vi "OSC_xuanshaowen.vi"() -> ()   [LabVIEW 2012]
uses:
  <vilib>/Utility/miscctls.llb/LVTextColorsTypeDef.ctl
  <vilib>/Utility/miscctls.llb/LVForegroundBackgroundColorsTypeDef.ctl
  GlobalVariable.vi
panel:
  in  "选项卡控件":T1(tab)
  in  "开始":bool
  in  "停止":bool
  in  "AutoScale":bool
  in  "sample mode":u16(ring)=10178 caption="Acquisition Mode" items=["有限采样"=10178, "连续采样"=10123]
  in  "TriggleSetting":T2={"Type"=enum."Immediate", "Source"="", "Horizontal Position (%)"=0.5, "slope"=10280, "level"=0.0} {"level" step=0.01 format="%0.2f"; "slope" items=["上升"=10280, "下降"=10171]; "Horizontal Position (%)" scale=0.0..1.0}
  in  "TimeBase":cluster{"Time/Div":dbl}={"Time/Div"=0.001} {"Time/Div" scale=5e-06..0.2}
  in  "Channel Setting 0":T3={"physical channels"="", "Enable"=TRUE, "Coupling"=enum."DC", "    Scale\n  Volts/Div  "=0.5, "    Vertical\nPosition (Div)"=0.0, "Meas Range"=10.0} {"Meas Range" items=["-0.1 V~+0.1 V"=0.1, "-0.2 V~0.2 V"=0.2, "-0.5 V~+0.5 V"=0.5, "-1 V~+1 V"=1.0, "-2 V~+2 V"=2.0, "-5 V~+5 V"=5.0, "-10 V~+10 V"=10.0]; "Vertical\nPosition (Div)" min=-5.0 max=5.0 step=0.01 scale=-5.0..5.0 scale format="%.2f"; "Scale\n  Volts/Div" scale=0.01..20.0}
  in  "Channel Setting 1":T3={"physical channels"="", "Enable"=FALSE, "Coupling"=enum."DC", "    Scale\n  Volts/Div  "=0.5, "    Vertical\nPosition (Div)"=0.0, "Meas Range"=10.0} {"Meas Range" items=["-0.1 V~+0.1 V"=0.1, "-0.2 V~0.2 V"=0.2, "-0.5 V~+0.5 V"=0.5, "-1 V~+1 V"=1.0, "-2 V~+2 V"=2.0, "-5 V~+5 V"=5.0, "-10 V~+10 V"=10.0]; "Vertical\nPosition (Div)" min=-5.0 max=5.0 step=0.01 scale=-5.0..5.0 scale format="%.2f"; "Scale\n  Volts/Div" scale=0.01..20.0}
  out "Some Information":T4={"设计者："="宣劭文（文少轩）", "指导教师："="侯成刚", "单位："="西安交通大学", "设计说明："="      该示波器是设计者的一门实验课程的大作业，分享仅作学习交流用，请勿用于商业用途，转载请说明出处，请务必保留原作信息。\n\n      示波器的性能指标是基于NI的ELVISmx而确定的，具体见附件中的设计说明文档。\n\n      如有问题，欢迎来信交流。\n", "联系方式："="swxuan@live.com"}
  out "SampleRate:":string
  in  "Cursors":T5={"Cursors On"=FALSE, "Cursor 1"=FALSE, "CurChan1 1"=0, "Cursor 2"=FALSE, "CurChan1 2"=1} {"CurChan1 2" items=["CH1", "CH2"]; "CurChan1 1" items=["CH1", "CH2"]}
  in  "Meas On/Off":cluster{"CH0 Meas":bool, "CH1 Meas":bool}
  out "Cursor":string
  out "CH1 Meas":string
  out "CH0 Meas":string
  out "波形图":waveform(dbl)[](graph)
  # "Trigger"
  # "Timebase"
  # "Channel 0 Settings"
  # "Channel 1 Settings"
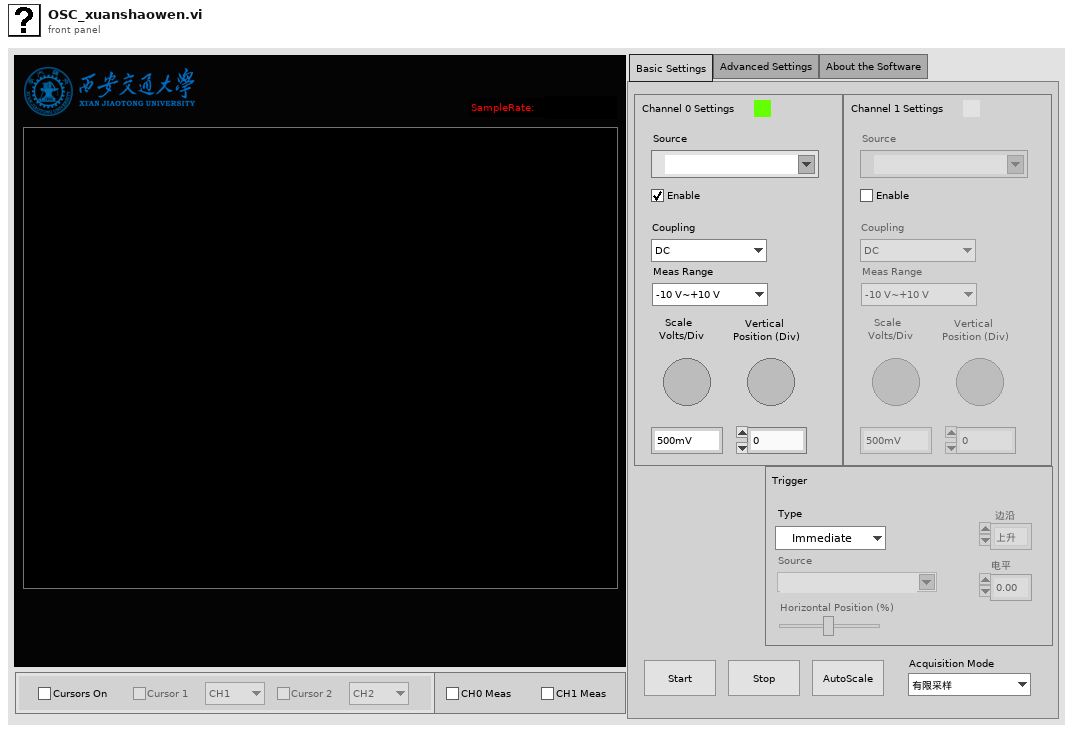
[diagram p1: front panel]
types:
  T1 = enum32{"Basic Settings", "Advanced Settings", "About the Software"}
  T2 = cluster{"Type":enum16{"Immediate", "Digital", "Edge"}, "Source":string, "Horizontal Position (%)":dbl, "slope":i32, "level":dbl}
  T3 = cluster{"physical channels":tag, "Enable":bool, "Coupling":enum16{"DC", "AC"}, "    Scale\n  Volts/Div  ":dbl, "    Vertical\nPosition (Div)":dbl, "Meas Range":dbl}
  T4 = cluster{"设计者：":string, "指导教师：":string, "单位：":string, "设计说明：":string, "联系方式：":string}
  T5 = cluster{"Cursors On":bool, "Cursor 1":bool, "CurChan1 1":u16, "Cursor 2":bool, "CurChan1 2":u16}
  T6 = typedef "LVForegroundBackgroundColorsTypeDef.ctl" = cluster{"Foreground Color":u32, "Background Color":u32}
  T7 = typedef "LVTextColorsTypeDef.ctl" = cluster{"Text Color":u32, "Background Color":u32}
  T8 = enum8{"Enabled", "Disabled", "Disabled and Grayed Out"}
  T9 = cluster{"数值输入控件":dbl, "最大值":dbl, "增量":dbl, "数值输入控件":dbl, "数值输入控件":dbl}
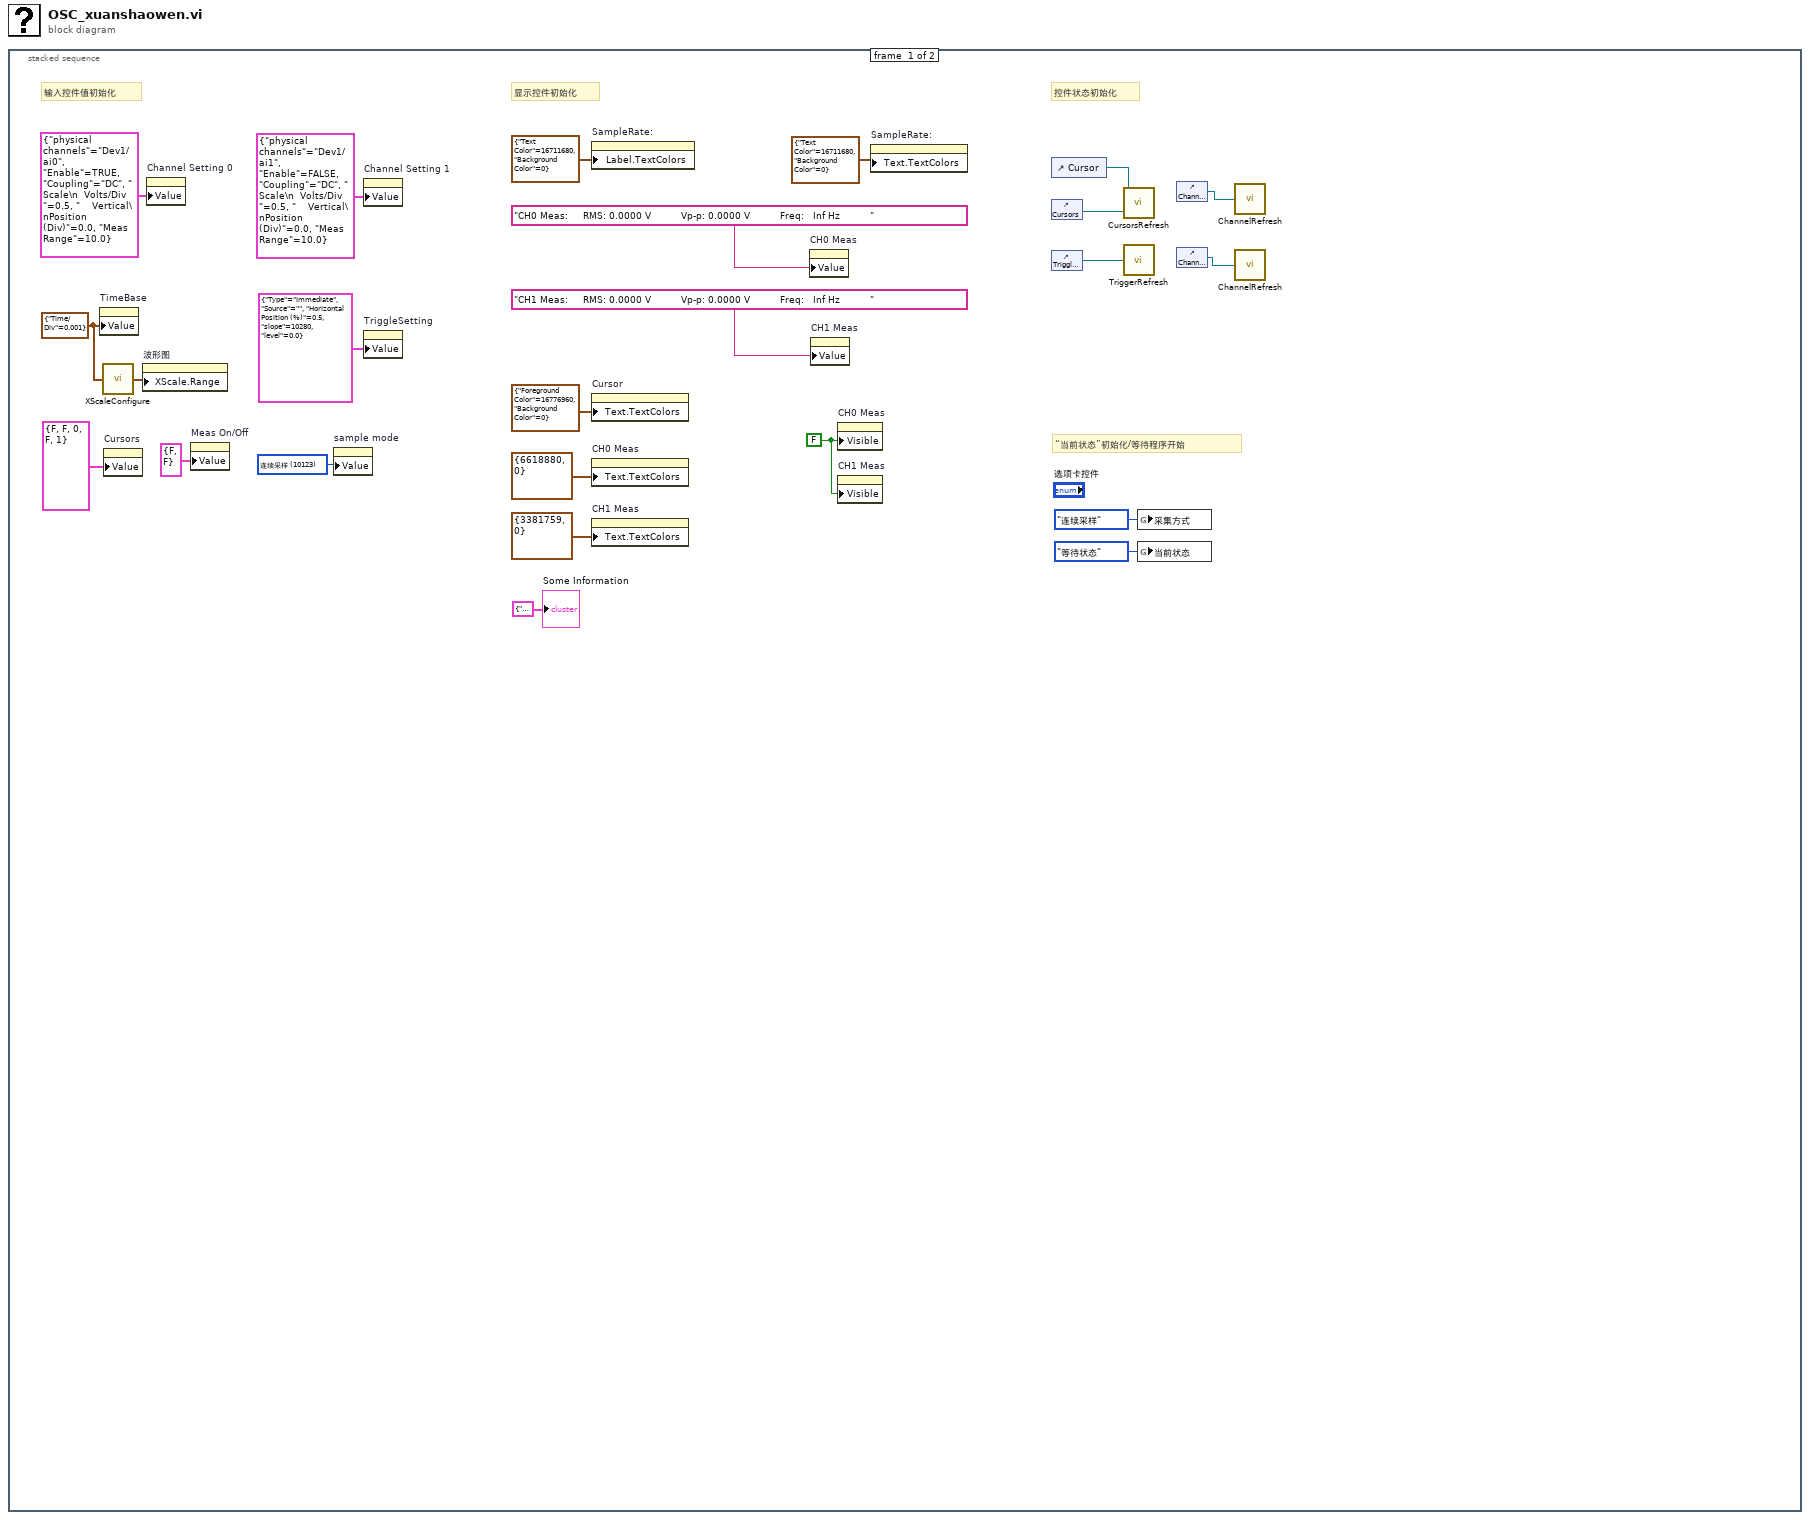
[diagram p0: block diagram]
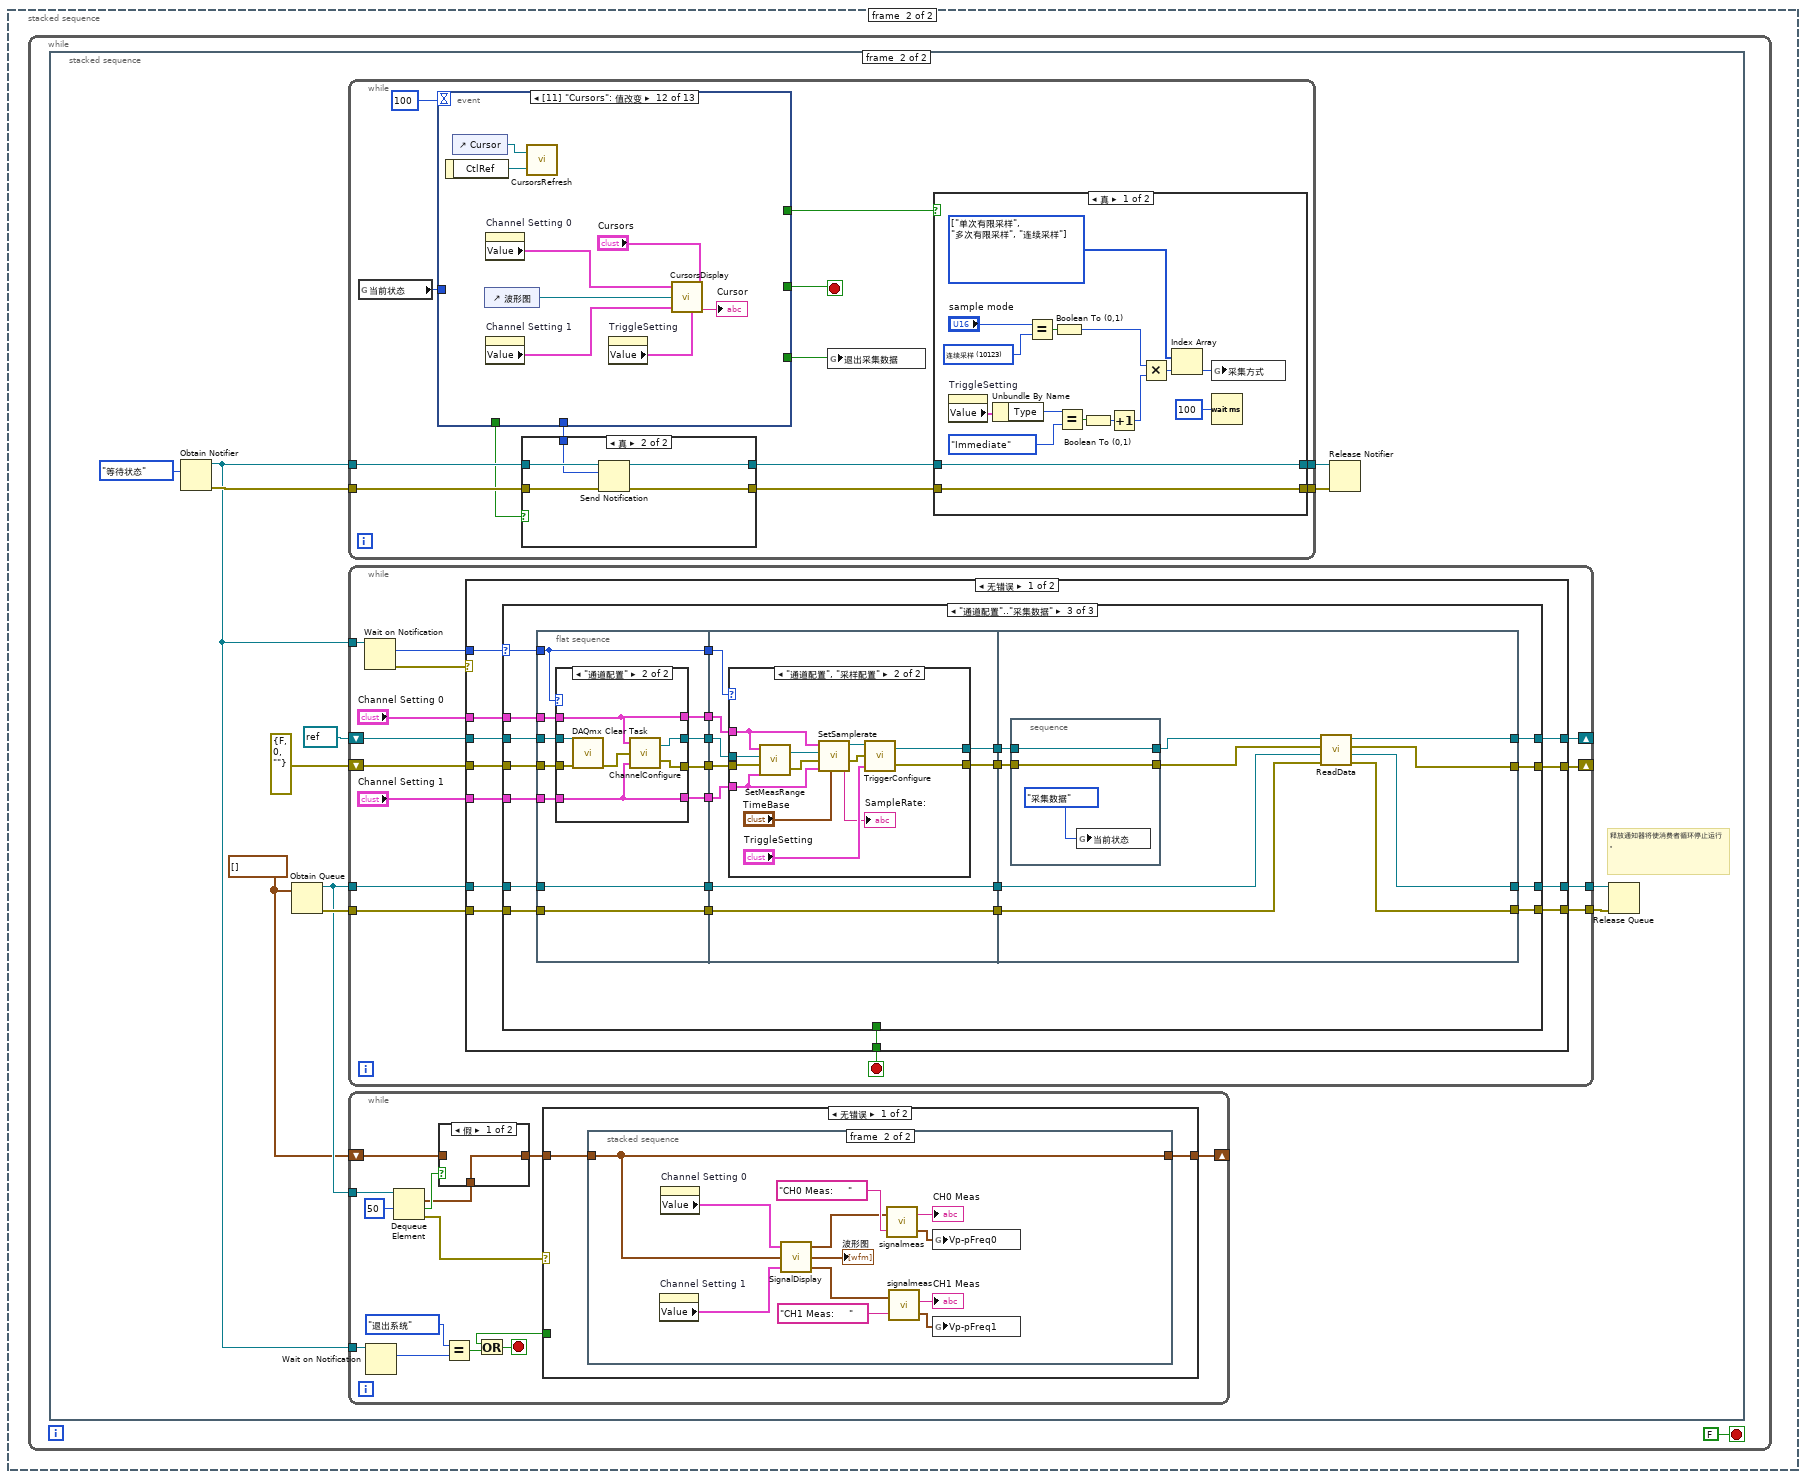
[diagram p2: hidden frame]
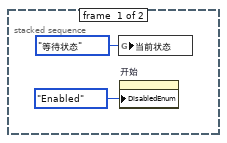
[diagram p3: hidden frame]
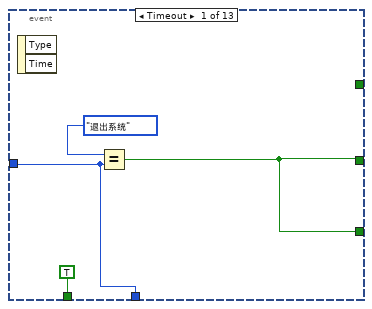
[diagram p5: hidden frame]
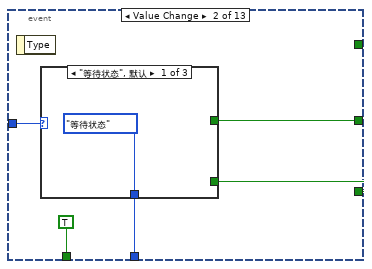
[diagram p6: hidden frame]
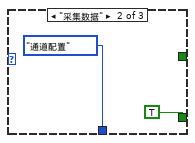
[diagram p7: hidden frame]
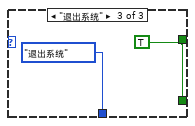
[diagram p8: hidden frame]
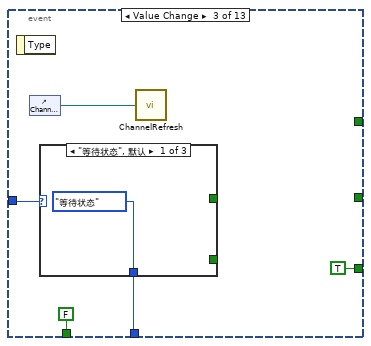
[diagram p9: hidden frame]
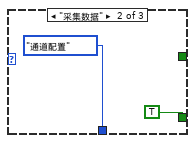
[diagram p10: hidden frame]
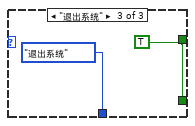
[diagram p11: hidden frame]
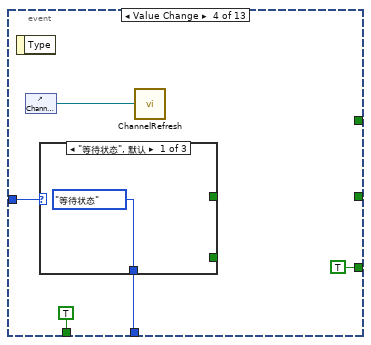
[diagram p12: hidden frame]
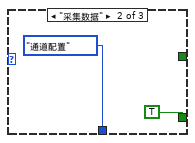
[diagram p13: hidden frame]
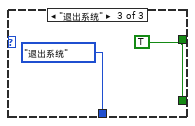
[diagram p14: hidden frame]
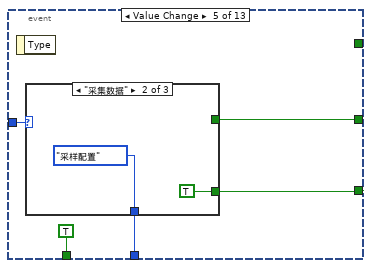
[diagram p15: hidden frame]
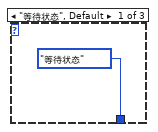
[diagram p16: hidden frame]
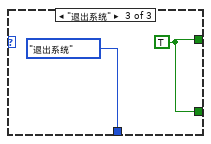
[diagram p17: hidden frame]
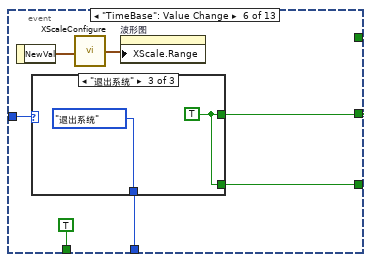
[diagram p18: hidden frame]
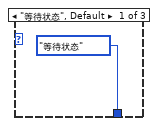
[diagram p19: hidden frame]
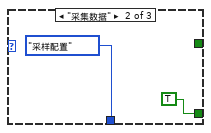
[diagram p20: hidden frame]
diagram:
  n1 = stacked-sequence {
    frame #0 {
      w2 = FALSE ("可见")
      w8 = u16 10123 items=["有限采样"=10178, "连续采样"=10123] ("sample mode")
      w22 = cluster{"Time/Div":dbl} {"Time/Div"=0.001} ("TimeBase")
      # "控件状态初始化"
      # "“当前状态”初始化/等待程序开始"
      # "显示控件初始化"
      # "输入控件值初始化"
      n2 = property on="TimeBase" class="Clust (严格)"("Value"=w22) -> ()  [unwired: 2 in, 2 out]
      n3 = call "XScaleConfigure.vi"("TimeBase"=w22) -> ("X坐标范围"=w21:T9)
      n4 = property on="Cursors" class="Clust (严格)"("Value"=T5 {"Cursors On"=FALSE, "Cursor 1"=FALSE, "CurChan1 1"=0, "Cursor 2"=FALSE, "CurChan1 2"=1} ("Cursors")) -> ()  [unwired: 2 in, 2 out]
      n5 = property on="波形图" class="WFGraph (严格)"("XScale.Range"=w21) -> ()  [unwired: 2 in, 2 out]
      n6 = property on="Channel Setting 0" class="Clust (严格)"("Value"=T3 {"physical channels"="Dev1/ai0", "Enable"=TRUE, "Coupling"=enum."DC", "    Scale\n  Volts/Div  "=0.5, "    Vertical\nPosition (Div)"=0.0, "Meas Range"=10.0} ("Channel Setting 0")) -> ()  [unwired: 2 in, 2 out]
      n7 = property on="Meas On/Off" class="Clust (严格)"("Value"=cluster{"CH0 Meas":bool, "CH1 Meas":bool} {"CH0 Meas"=FALSE, "CH1 Meas"=FALSE} ("Meas On/Off")) -> ()  [unwired: 2 in, 2 out]
      n8 = property on="sample mode" class="Ring (严格)"("Value"=w8) -> ()  [unwired: 2 in, 2 out]
      n9 = property on="Channel Setting 1" class="Clust (严格)"("Value"=T3 {"physical channels"="Dev1/ai1", "Enable"=FALSE, "Coupling"=enum."DC", "    Scale\n  Volts/Div  "=0.5, "    Vertical\nPosition (Div)"=0.0, "Meas Range"=10.0} ("Channel Setting 0")) -> ()  [unwired: 2 in, 2 out]
      n10 = property on="TriggleSetting" class="Clust (严格)"("Value"=T2 {"Type"=enum."Immediate", "Source"="", "Horizontal Position (%)"=0.5, "slope"=10280, "level"=0.0} ("TriggleSetting")) -> ()  [unwired: 2 in, 2 out]
      n11 = property on="SampleRate:" class="Str"("Label.TextColors"=T7 {"Text Color"=16711680, "Background Color"=0} ("标签.文本颜色")) -> ()  [unwired: 2 in, 2 out]
      n12 = property on="Cursor" class="Str"("Text.TextColors"=T6 {"Foreground Color"=16776960, "Background Color"=0} ("文本.颜色")) -> ()  [unwired: 2 in, 2 out]
      n13 = property on="CH0 Meas" class="Str"("Text.TextColors"=T7 {"Text Color"=6618880, "Background Color"=0} ("文本.文本颜色")) -> ()  [unwired: 2 in, 2 out]
      n14 = property on="CH1 Meas" class="Str"("Text.TextColors"=T7 {"Text Color"=3381759, "Background Color"=0} ("文本.文本颜色")) -> ()  [unwired: 2 in, 2 out]
      n15 = property on="CH0 Meas" class="Str"("Value"="CH0 Meas:     RMS: 0.0000 V          Vp-p: 0.0000 V          Freq:   Inf Hz          " ("CH0 Meas")) -> ()  [unwired: 2 in, 2 out]
      n16 = property on="CH1 Meas" class="Str"("Value"="CH1 Meas:     RMS: 0.0000 V          Vp-p: 0.0000 V          Freq:   Inf Hz          " ("CH1 Meas")) -> ()  [unwired: 2 in, 2 out]
      n17 = property on="CH0 Meas" class="Str"("Visible"=w2) -> ()  [unwired: 2 in, 2 out]
      n18 = property on="CH1 Meas" class="Str"("Visible"=w2) -> ()  [unwired: 2 in, 2 out]
      n19 = property on="SampleRate:" class="Str"("Text.TextColors"=T7 {"Text Color"=16711680, "Background Color"=0} ("数值文本.文本颜色")) -> ()  [unwired: 2 in, 2 out]
      n20 = control-ref of="Cursor"() -> (w9:refnum<vi>)
      n21 = control-ref of="Cursors"() -> (w10:refnum<vi>)
      n22 = control-ref of="TriggleSetting"() -> (w7:refnum<vi>)
      n23 = call "CursorsRefresh.vi"("Cursors簇句柄引用"=w10, "Cursor字符串句柄引用"=w9) -> ()  [unwired: 2 in]
      n24 = call "TriggerRefresh.vi"("TriggerSetting引用句柄"=w7) -> ()
      n25 = global write "GlobalVariable.vi" "采集方式"(enum16{"单次有限采样", "多次有限采样", "连续采样"}."连续采样" ("采集方式")) -> ()
      n26 = global write "GlobalVariable.vi" "当前状态"(enum16{"等待状态", "采集数据", "退出系统"}."等待状态" ("当前状态")) -> ()
      n27 = control-ref of="Channel Setting 0"() -> (w6:refnum<vi>)
      n28 = control-ref of="Channel Setting 1"() -> (w5:refnum<vi>)
      n29 = call "ChannelRefresh.vi"("Channel Setting 引用句柄"=w6) -> ()
      n30 = call "ChannelRefresh.vi"("Channel Setting 引用句柄"=w5) -> ()
      "Some Information" <- T4 {"设计者："="宣劭文（文少轩）", "指导教师："="侯成刚", "单位："="西安交通大学", "设计说明："="      该示波器是设计者的一门实验课程的大作业，分享仅作学习交流用，请勿用于商业用途，转载请说明出处，请务必保留原作信息。\n\n      示波器的性能指标是基于NI的ELVISmx而确定的，具体见附件中的设计说明文档。\n\n      如有问题，欢迎来信交流。\n", "联系方式："="swxuan@live.com"} ("Some Information")
    }
    frame #1 {
      n31 = while {
        stop <- FALSE stop-if-true
        n32 = stacked-sequence {
          frame #0 {
            n33 = global write "GlobalVariable.vi" "当前状态"(enum16{"等待状态", "采集数据", "退出系统"}."等待状态" ("当前状态")) -> ()
            n34 = property on="开始" class="Bool"("DisabledEnum"=T8."Enabled" ("禁用")) -> ()  [unwired: 2 in, 2 out]
          }
          frame #1 {
            w28 = waveform(dbl)[] [] ("data")
            # "释放通知器将使消费者循环停止运行。"
            n35 = Obtain Notifier(notification data type=enum16{"等待状态", "通道配置", "采样配置", "采集数据", "退出系统"}."等待状态" ("当前状态")) -> (notifier out=w31:refnum<notifier>, error out=w35:errorcluster)  [unwired: 2 in, 2 out]
            n36 = Obtain Queue(element data type=w28) -> (queue out=w36:refnum<queue>, error out=w39:errorcluster)  [unwired: 4 in, 1 out]
            n37 = while {
              tunnel: w31 -> [w52]
              tunnel: w35 -> [w51]
              tunnel: [w48] -> w34
              tunnel: [w47] -> w33
              stop <- w42 stop-if-true
              n38 = global read "GlobalVariable.vi" "当前状态"() -> (w46:enum16{"等待状态", "采集数据", "退出系统"})
              n39 = event shown="[11] \"Cursors\": 值改变" {
                selector: _ -> [_ _ _ _ _ _ _ _ _ _ _ _ _]
                dyn-events: _ -> [_ _ _ _ _ _ _ _ _ _ _ _ _]
                timeout: 100 -> [_ _ _ _ _ _ _ _ _ _ _ _ _]
                tunnel: w46 -> [w72 w79 w86 w96 w109 w120 w132 _ _ w149 w166 _ _]
                tunnel: [w72 w78 w85 w95 w108 w119 w131 enum16{"等待状态", "通道配置", "采样配置", "采集数据", "退出系统"}."通道配置" ("当前状态") enum16{"等待状态", "通道配置", "采样配置", "采集数据", "退出系统"}."退出系统" ("当前状态") w147 w165 _ _] -> w44
                tunnel: [TRUE TRUE FALSE TRUE TRUE TRUE TRUE TRUE TRUE w148 TRUE _ _] -> w43
                tunnel: [w71 w76 _ _ w106 w117 w129 _ w142 w145 w163 _ _] -> w42
                tunnel: [w71 w75 TRUE TRUE w105 w115 w128 _ w142 w146 w162 _ _] -> w41
                tunnel: [_ _ _ _ _ _ TRUE _ _ _ TRUE _ _] -> w40
                event Timeout {
                  n40 = event-data() -> ()  [unwired: 1 in, 2 out]
                  n41 = Equal?(x=enum16{"等待状态", "采集数据", "退出系统"}."退出系统", y=w72) -> (x = y?=w71:bool)
                }
                event "Channel Setting 0.physical channels", "Channel Setting 1.physical channels": Value Change {
                  n42 = event-data() -> ()  [unwired: 1 in, 1 out]
                  n43 = case shown="\"等待状态\", 默认" w79 {
                    tunnel: [enum16{"等待状态", "通道配置", "采样配置", "采集数据", "退出系统"}."等待状态" ("当前状态") enum16{"等待状态", "通道配置", "采样配置", "采集数据", "退出系统"}."通道配置" ("当前状态") enum16{"等待状态", "通道配置", "采样配置", "采集数据", "退出系统"}."退出系统" ("当前状态")] -> w78
                    tunnel: [_ TRUE w83] -> w75
                    tunnel: [_ _ w83] -> w76
                    frame "等待状态", Default {
                    }
                    frame "采集数据" {
                    }
                    frame "退出系统" {
                      w83 = TRUE
                    }
                  }
                }
                event "Channel Setting 0.Enable": Value Change {
                  n44 = event-data() -> ()  [unwired: 1 in, 1 out]
                  n45 = control-ref of="Channel Setting 0"() -> (w89:refnum<vi>)
                  n46 = case shown="\"等待状态\", 默认" w86 {
                    tunnel: [enum16{"等待状态", "通道配置", "采样配置", "采集数据", "退出系统"}."等待状态" ("当前状态") enum16{"等待状态", "通道配置", "采样配置", "采集数据", "退出系统"}."通道配置" ("当前状态") enum16{"等待状态", "通道配置", "采样配置", "采集数据", "退出系统"}."退出系统" ("当前状态")] -> w85
                    tunnel: [_ TRUE w93] -> _
                    tunnel: [_ _ w93] -> _
                    frame "等待状态", Default {
                    }
                    frame "采集数据" {
                    }
                    frame "退出系统" {
                      w93 = TRUE
                    }
                  }
                  n47 = call "ChannelRefresh.vi"("Channel Setting 引用句柄"=w89) -> ()
                }
                event "Channel Setting 1.Enable": Value Change {
                  n48 = event-data() -> ()  [unwired: 1 in, 1 out]
                  n49 = control-ref of="Channel Setting 1"() -> (w99:refnum<vi>)
                  n50 = case shown="\"等待状态\", 默认" w96 {
                    tunnel: [enum16{"等待状态", "通道配置", "采样配置", "采集数据", "退出系统"}."等待状态" ("当前状态") enum16{"等待状态", "通道配置", "采样配置", "采集数据", "退出系统"}."通道配置" ("当前状态") enum16{"等待状态", "通道配置", "采样配置", "采集数据", "退出系统"}."退出系统" ("当前状态")] -> w95
                    tunnel: [_ TRUE w103] -> _
                    tunnel: [_ _ w103] -> _
                    frame "等待状态", Default {
                    }
                    frame "采集数据" {
                    }
                    frame "退出系统" {
                      w103 = TRUE
                    }
                  }
                  n51 = call "ChannelRefresh.vi"("Channel Setting 引用句柄"=w99) -> ()
                }
                event "Channel Setting 0.Meas Range", "Channel Setting 1.Meas Range": Value Change {
                  n52 = event-data() -> ()  [unwired: 1 in, 1 out]
                  n53 = case shown="\"采集数据\"" w109 {
                    tunnel: [enum16{"等待状态", "通道配置", "采样配置", "采集数据", "退出系统"}."等待状态" ("当前状态") enum16{"等待状态", "通道配置", "采样配置", "采集数据", "退出系统"}."采样配置" ("当前状态") enum16{"等待状态", "通道配置", "采样配置", "采集数据", "退出系统"}."退出系统" ("当前状态")] -> w108
                    tunnel: [_ TRUE w114] -> w105
                    tunnel: [_ _ w114] -> w106
                    frame "等待状态", Default {
                    }
                    frame "采集数据" {
                    }
                    frame "退出系统" {
                      w114 = TRUE
                    }
                  }
                }
                event "TimeBase": Value Change {
                  n54 = event-data() -> ("NewVal"=w121:cluster{"Time/Div":dbl})  [unwired: 1 in]
                  n55 = case shown="\"退出系统\"" w120 {
                    tunnel: [enum16{"等待状态", "通道配置", "采样配置", "采集数据", "退出系统"}."等待状态" ("当前状态") enum16{"等待状态", "通道配置", "采样配置", "采集数据", "退出系统"}."采样配置" ("当前状态") enum16{"等待状态", "通道配置", "采样配置", "采集数据", "退出系统"}."退出系统" ("当前状态")] -> w119
                    tunnel: [_ _ w125] -> w117
                    tunnel: [_ TRUE w125] -> w115
                    frame "等待状态", Default {
                    }
                    frame "采集数据" {
                    }
                    frame "退出系统" {
                      w125 = TRUE
                    }
                  }
                  n56 = call "XScaleConfigure.vi"("TimeBase"=w121) -> ("X坐标范围"=w116:T9)
                  n57 = property on="波形图" class="WFGraph (严格)"("XScale.Range"=w116) -> ()  [unwired: 2 in, 2 out]
                }
                event "TriggleSetting": Value Change {
                  n58 = event-data() -> ("CtlRef"=w133:refnum<vi>)  [unwired: 1 in]
                  n59 = case shown="\"退出系统\"" w132 {
                    tunnel: [enum16{"等待状态", "通道配置", "采样配置", "采集数据", "退出系统"}."等待状态" ("当前状态") enum16{"等待状态", "通道配置", "采样配置", "采集数据", "退出系统"}."采样配置" ("当前状态") enum16{"等待状态", "通道配置", "采样配置", "采集数据", "退出系统"}."退出系统" ("当前状态")] -> w131
                    tunnel: [_ TRUE w137] -> w128
                    tunnel: [_ _ w137] -> w129
                    frame "等待状态", Default {
                    }
                    frame "采集数据" {
                    }
                    frame "退出系统" {
                      w137 = TRUE
                    }
                  }
                  n60 = call "TriggerRefresh.vi"("TriggerSetting引用句柄"=w133) -> ()
                }
                event "开始": Value Change {
                  n61 = event-data() -> ()  [unwired: 1 in, 1 out]
                  n62 = property on="开始" class="Bool"("DisabledEnum"=T8."Disabled and Grayed Out" ("禁用")) -> ()  [unwired: 2 in, 2 out]
                }
                event "停止": Value Change {
                  w142 = TRUE
                  n63 = event-data() -> ()  [unwired: 1 in, 1 out]
                }
                event "AutoScale": Value Change {
                  n64 = event-data() -> ()  [unwired: 1 in, 1 out]
                  n65 = case shown="\"采集数据\"" w149 {
                    tunnel: [_ _ w158] -> w145
                    tunnel: [_ enum16{"等待状态", "通道配置", "采样配置", "采集数据", "退出系统"}."采样配置" ("当前状态") enum16{"等待状态", "通道配置", "采样配置", "采集数据", "退出系统"}."退出系统" ("当前状态")] -> w147
                    tunnel: [_ TRUE TRUE] -> w148
                    tunnel: [_ TRUE w158] -> w146
                    frame "等待状态", Default {
                    }
                    frame "采集数据" {
                      n66 = property on="Enable" class="Bool (严格)"() -> ("Value"=w157:bool)  [unwired: 2 in, 2 out]
                      n67 = property on="Enable" class="Bool (严格)"() -> ("Value"=w156:bool)  [unwired: 2 in, 2 out]
                      n68 = call "AutoScale.vi"("Channel 1 Enable"=w156, "Channel 0 Enable"=w157) -> ("Scale\n  Volts/Div 1"=w153:dbl, "Time/Div"=w154:dbl, "Scale\n  Volts/Div 0"=w155:dbl)  [unwired: 2 in]
                      n69 = property on="Time/Div" class="Knob (严格)"("Value"=w154) -> ()  [unwired: 2 in, 2 out]
                      n70 = property on="Scale\n  Volts/Div" class="Knob (严格)"("Value"=w155) -> ()  [unwired: 2 in, 2 out]
                      n71 = property on="Scale\n  Volts/Div" class="Knob (严格)"("Value"=w153) -> ()  [unwired: 2 in, 2 out]
                    }
                    frame "退出系统" {
                      w158 = TRUE
                    }
                  }
                }
                event "sample mode": Value Change {
                  n72 = event-data() -> ()  [unwired: 1 in, 1 out]
                  n73 = case shown="\"等待状态\", 默认" w166 {
                    tunnel: [enum16{"等待状态", "通道配置", "采样配置", "采集数据", "退出系统"}."等待状态" ("当前状态") enum16{"等待状态", "通道配置", "采样配置", "采集数据", "退出系统"}."采样配置" ("当前状态") enum16{"等待状态", "通道配置", "采样配置", "采集数据", "退出系统"}."退出系统" ("当前状态")] -> w165
                    tunnel: [_ TRUE w170] -> w162
                    tunnel: [_ _ w170] -> w163
                    frame "等待状态", Default {
                    }
                    frame "采集数据" {
                    }
                    frame "退出系统" {
                      w170 = TRUE
                    }
                  }
                }
                event "Cursors": Value Change {
                  n74 = event-data() -> ("CtlRef"=w179:refnum<vi>)  [unwired: 1 in]
                  n75 = control-ref of="Cursor"() -> (w178:refnum<vi>)
                  n76 = control-ref of="波形图"() -> (w176:refnum<vi>)
                  n77 = property on="Channel Setting 0" class="Clust (严格)"() -> ("Value"=w177:T3)  [unwired: 2 in, 2 out]
                  n78 = property on="Channel Setting 1" class="Clust (严格)"() -> ("Value"=w175:T3)  [unwired: 2 in, 2 out]
                  n79 = call "CursorsRefresh.vi"("Cursors簇句柄引用"=w179, "Cursor字符串句柄引用"=w178) -> ()  [unwired: 2 in]
                  n80 = property on="TriggleSetting" class="Clust (严格)"() -> ("Value"=w174:T2)  [unwired: 2 in, 2 out]
                  n81 = call "CursorsDisplay.vi"("Channel Setting 0"=w177, "波形图引用句柄"=w176, "Channel Setting 1"=w175, "Cursors"="Cursors", "TriggleSetting"=w174) -> ("Cursor"=→"Cursor":string)  [unwired: 5 in]
                }
                event "Meas On/Off": Value Change {
                  n82 = event-data() -> ("NewVal"=w180:cluster{"CH0 Meas":bool, "CH1 Meas":bool})  [unwired: 1 in]
                  n83 = Unbundle By Name(w180) -> ("CH0 Meas"=w181:bool, "CH1 Meas"=w182:bool)
                  n84 = property on="CH1 Meas" class="Str"("Visible"=w182) -> ()  [unwired: 2 in, 2 out]
                  n85 = property on="CH0 Meas" class="Str"("Visible"=w181) -> ()  [unwired: 2 in, 2 out]
                }
              }
              n86 = case shown="真" w43 {
                tunnel: w52 -> [w183 w189]
                tunnel: [w184 w188] -> w49
                tunnel: w51 -> [w184 w187]
                tunnel: [w183 w186] -> w50
                tunnel: w44 -> [_ w185]
                frame False {
                }
                frame True {
                  n87 = Send Notification(notification=w185, notifier=w189, error in (no error)=w187) -> (notifier out=w186:refnum<notifier>, error out=w188:errorcluster)
                }
              }
              n88 = global write "GlobalVariable.vi" "退出采集数据"(w41) -> ()
              n89 = case shown="真" w40 {
                tunnel: w50 -> [w57 w70]
                tunnel: w49 -> [w56 w69]
                tunnel: [w57 w70] -> w48
                tunnel: [w56 w69] -> w47
                frame True {
                  w59 = u16 10123 items=["有限采样"=10178, "连续采样"=10123] ("sample mode")
                  w68 = enum16{"单次有限采样", "多次有限采样", "连续采样"}[] [enum."单次有限采样", enum."多次有限采样", enum."连续采样"] items=["单次有限采样", "多次有限采样", "连续采样"]
                  n90 = property on="TriggleSetting" class="Clust (严格)"() -> ("Value"=w63:T2)  [unwired: 2 in, 2 out]
                  n91 = Unbundle By Name(w63) -> ("Type"=w62:enum16{"Immediate", "Digital", "Edge"})
                  n92 = Equal?(x="sample mode", y=w59) -> (x = y?=w60:bool)
                  n93 = Boolean To (0,1)(Boolean=w60) -> (0, 1=w67:i16)
                  n94 = Equal?(x=w62, y=enum16{"Immediate", "Digital", "Edge"}."Immediate") -> (x = y?=w64:bool)
                  n95 = Boolean To (0,1)(Boolean=w64) -> (0, 1=w65:i16)
                  n96 = Increment(x=w65) -> (x+1=w66:i16)
                  n97 = Multiply(x=w67, y=w66) -> (x*y=w54:i16)
                  n98 = Index Array(array=w68, index=w54) -> (element=w55:enum16{"单次有限采样", "多次有限采样", "连续采样"})
                  n99 = global write "GlobalVariable.vi" "采集方式"(w55) -> ()
                  n100 = Wait (ms)(milliseconds to wait=u32 100 ("等待时间（毫秒）")) -> ()  [unwired: 1 out]
                }
                frame False {
                }
              }
            }
            n101 = while {
              tunnel: w36 -> [w241]
              tunnel: w39 -> [w240]
              tunnel: [w239] -> w38
              tunnel: [w238] -> w37
              tunnel: w31 -> [w237]
              shift-right: [w233] -> _
              shift-left: refnum<k21> refnum ("task out") -> [w234]
              shift-right: [w235] -> _
              shift-left: errorcluster {"status"=FALSE, "code"=0, "source"=""} ("error out") -> [w236]
              stop <- w230 stop-if-true
              n102 = Wait on Notification(notifier=w237) -> (notification=w232:enum16{"等待状态", "通道配置", "采样配置", "采集数据", "退出系统"}, error out=w231:errorcluster)  [unwired: 1 in, 4 out]
              n103 = case shown="无错误" w231 {
                tunnel: w241 -> [w253 w350]
                tunnel: w240 -> [w252 w349]
                tunnel: [w251 w350] -> w239
                tunnel: [w250 w349] -> w238
                tunnel: w236 -> [w249 w347]
                tunnel: [w248 w347] -> w235
                tunnel: w234 -> [w247 w348]
                tunnel: [w246 w348] -> w233
                tunnel: w232 -> [w244 _]
                tunnel: [w245 TRUE] -> w230
                tunnel: "Channel Setting 0" -> [w243 _]
                tunnel: "Channel Setting 1" -> [w242 _]
                frame No Error {
                  n104 = case shown="\"通道配置\"..\"采集数据\"" w244 {
                    selector: w244 -> [_ _ w286]
                    tunnel: w253 -> [w256 w261 w283]
                    tunnel: w252 -> [w255 w260 w282]
                    tunnel: [w256 w261 w281] -> w251
                    tunnel: [w255 w260 w280] -> w250
                    tunnel: w249 -> [w257 w262 w284]
                    tunnel: [w257 w262 w278] -> w248
                    tunnel: w247 -> [w258 w263 w285]
                    tunnel: [w258 w263 w279] -> w246
                    tunnel: [_ TRUE _] -> w245
                    tunnel: w243 -> [_ _ w271]
                    tunnel: w242 -> [_ _ w270]
                    frame "等待状态", Default {
                      n105 = Wait (ms)(milliseconds to wait=u32 50 ("等待时间（毫秒）")) -> ()  [unwired: 1 out]
                    }
                    frame "退出系统" {
                      n106 = global write "GlobalVariable.vi" "当前状态"(enum16{"等待状态", "采集数据", "退出系统"}."退出系统" ("当前状态")) -> ()
                    }
                    frame "通道配置".."采集数据" {
                      n107 = flat-sequence {
                        tunnel: w286 -> [w287]
                        tunnel: w285 -> [w297]
                        tunnel: [w293] -> w277
                        tunnel: w284 -> [w296]
                        tunnel: [w292] -> w276
                        tunnel: w283 -> [w295]
                        tunnel: [w295] -> w275
                        tunnel: w282 -> [w294]
                        tunnel: [w294] -> w274
                        tunnel: w271 -> [w291]
                        tunnel: w270 -> [w290]
                        tunnel: [w289] -> w269
                        tunnel: [w288] -> w268
                        tunnel: [w287] -> w267
                        tunnel: w277 -> [w317]
                        tunnel: w276 -> [w316]
                        tunnel: w275 -> [w315]
                        tunnel: [w315] -> w273
                        tunnel: w274 -> [w314]
                        tunnel: [w314] -> w272
                        tunnel: w269 -> [w313]
                        tunnel: w268 -> [w312]
                        tunnel: w267 -> [w311]
                        tunnel: [w310] -> w266
                        tunnel: [w309] -> w265
                        tunnel: w273 -> [w336]
                        tunnel: w272 -> [w335]
                        tunnel: [w334] -> w281
                        tunnel: [w333] -> w280
                        tunnel: [w340] -> w279
                        tunnel: [w339] -> w278
                        tunnel: w266 -> [w338]
                        tunnel: w265 -> [w337]
                        frame #0 {
                          n108 = case shown="\"通道配置\"" w287 {
                            tunnel: w297 -> [w301 w307]
                            tunnel: w296 -> [w300 w306]
                            tunnel: [w301 w305] -> w293
                            tunnel: [w300 w304] -> w292
                            tunnel: w291 -> [w299 w303]
                            tunnel: w290 -> [w298 w302]
                            tunnel: [w299 w303] -> w289
                            tunnel: [w298 w302] -> w288
                            frame "采样配置", "采集数据", Default {
                            }
                            frame "通道配置" {
                              n109 = call <vilib>:"DAQmx Clear Task.vi"("task in"=w307, "error in"=w306) -> ("error out"=w308:errorcluster)  [unwired: 13 in]
                              n110 = call "ChannelConfigure.vi"("Channel Setting 1"=w302, "Error In"=w308, "Channel Setting 0"=w303) -> ("Error Out"=w304:errorcluster, "Task Out"=w305:refnum<k21>)
                            }
                          }
                        }
                        frame #1 {
                          n111 = case shown="\"通道配置\", \"采样配置\"" w311 {
                            tunnel: w317 -> [w319 w328]
                            tunnel: w316 -> [w318 w327]
                            tunnel: w313 -> [_ w326]
                            tunnel: w312 -> [_ w325]
                            tunnel: [w319 w321] -> w310
                            tunnel: [w318 w320] -> w309
                            frame "采集数据", Default {
                            }
                            frame "通道配置", "采样配置" {
                              n112 = call "SetMeasRange.vi"("Channel Setting 1"=w325, "Error In"=w327, "Task In"=w328, "Channel Setting 0"=w326) -> ("Error Out"=w330:errorcluster, "Task Out"=w331:refnum<k21>)
                              n113 = call "SetSamplerate.vi"("TimeBase"="TimeBase", "Channel Setting 1"=w325, "Error In"=w330, "Task In"=w331, "Channel Setting 0"=w326) -> ("采样率"=→"SampleRate:":string, "Error Out"=w322:errorcluster, "Task Out"=w323:refnum<k21>)  [unwired: 2 in]
                              n114 = call "TriggerConfigure.vi"("TriggleSetting"="TriggleSetting", "Error In"=w322, "Task In"=w323) -> ("Error Out"=w320:errorcluster, "Task Out"=w321:refnum<k21>)
                            }
                          }
                        }
                        frame #2 {
                          n115 = stacked-sequence {
                            tunnel: [w345] -> w341
                            tunnel: w338 -> [w345]
                            tunnel: [w344] -> w342
                            tunnel: w337 -> [w344]
                            frame #0 {
                              n116 = global write "GlobalVariable.vi" "当前状态"(enum16{"等待状态", "采集数据", "退出系统"}."采集数据" ("当前状态")) -> ()
                            }
                          }
                          n117 = call "ReadData.vi"("错误输入（队列）"=w335, "队列输入"=w336, "错误输入（采集）"=w342, "Task In"=w341) -> ("错误输出（队列）"=w333:errorcluster, "队列输出"=w334:refnum<queue>, "错误输出（采集）"=w339:errorcluster, "Task Out"=w340:refnum<k21>)
                        }
                      }
                    }
                  }
                }
                frame Error {
                  n118 = global write "GlobalVariable.vi" "当前状态"(enum16{"等待状态", "采集数据", "退出系统"}."退出系统" ("当前状态")) -> ()
                }
              }
            }
            n119 = while {
              tunnel: w36 -> [w203]
              tunnel: w31 -> [w200]
              shift-right: [w190] -> _
              shift-left: w28 -> [w193]
              stop <- w202 stop-if-true
              n120 = Wait on Notification(notifier=w200) -> (notification=w198:enum16{"等待状态", "通道配置", "采样配置", "采集数据", "退出系统"})  [unwired: 1 in, 5 out]
              n121 = Dequeue Element(queue=w203, timeout in ms (-1)=50 ("超时毫秒(-1)")) -> (element=w192:waveform(dbl)[], timed out?=w194:bool, error out=w197:errorcluster)  [unwired: 1 in, 1 out]
              n122 = case shown="假" w194 {
                tunnel: w193 -> [_ w205]
                tunnel: w192 -> [w204 _]
                tunnel: [w204 w205] -> w191
                frame False {
                }
                frame True {
                }
              }
              n123 = Equal?(x=enum16{"等待状态", "通道配置", "采样配置", "采集数据", "退出系统"}."退出系统" ("当前状态"), y=w198) -> (x = y?=w201:bool)
              n124 = case shown="无错误" w197 {
                tunnel: [_ TRUE] -> w196
                tunnel: w191 -> [w207 _]
                tunnel: [w206 _] -> w190
                frame No Error {
                  n125 = stacked-sequence {
                    tunnel: w207 -> [_ w214]
                    tunnel: [_ w214] -> w206
                    frame #0 {
                      n126 = property on="Channel Setting 0" class="Clust (严格)"() -> ("Value"=w213:T3)  [unwired: 2 in, 2 out]
                      n127 = control-ref of="波形图"() -> (w211:refnum<vi>)
                      n128 = property on="Channel Setting 1" class="Clust (严格)"() -> ("Value"=w212:T3)  [unwired: 2 in, 2 out]
                      n129 = property on="TriggleSetting" class="Clust (严格)"() -> ("Value"=w208:T2)  [unwired: 2 in, 2 out]
                      n130 = property on="Cursors" class="Clust (严格)"() -> ("Value"=w209:T5)  [unwired: 2 in, 2 out]
                      n131 = call "CursorsDisplay.vi"("Channel Setting 0"=w213, "波形图引用句柄"=w211, "Channel Setting 1"=w212, "Cursors"=w209, "TriggleSetting"=w208) -> ("Cursor"=w210:string)  [unwired: 5 in]
                      n132 = property on="Cursor" class="Str"("Value"=w210) -> ()  [unwired: 2 in, 2 out]
                    }
                    frame #1 {
                      n133 = property on="Channel Setting 1" class="Clust (严格)"() -> ("Value"=w220:T3)  [unwired: 2 in, 2 out]
                      n134 = property on="Channel Setting 0" class="Clust (严格)"() -> ("Value"=w221:T3)  [unwired: 2 in, 2 out]
                      n135 = call "SignalDisplay.vi"("Channel Setting 1"=w220, "Double_Channel_Data_In"=w214, "Channel Setting 0"=w221) -> ("Data_for_measure_out 1"=w223:waveform(dbl), "波形图"=→"波形图":waveform(dbl)[], "Data_for_measure_out 0"=w222:waveform(dbl))
                      n136 = call "signalmeas.vi"("前缀"="CH0 Meas:     " ("字符串"), "Data In"=w222) -> ("Vp-pFreq"=w217:cluster{"Vp-p":dbl, "detected frequency":dbl}, "测量字符串"=→"CH0 Meas":string)
                      n137 = call "signalmeas.vi"("前缀"="CH1 Meas:     " ("字符串"), "Data In"=w223) -> ("Vp-pFreq"=w216:cluster{"Vp-p":dbl, "detected frequency":dbl}, "测量字符串"=→"CH1 Meas":string)
                      n138 = global write "GlobalVariable.vi" "Vp-pFreq0"(w217) -> ()
                      n139 = global write "GlobalVariable.vi" "Vp-pFreq1"(w216) -> ()
                    }
                  }
                }
                frame Error {
                  # "当错误发生时，返回\n真，停止程序"
                  n140 = global write "GlobalVariable.vi" "当前状态"(enum16{"等待状态", "采集数据", "退出系统"}."退出系统" ("当前状态")) -> ()
                }
              }
              n141 = Or(x=w196, y=w201) -> (x .or. y?=w202:bool)
            }
            n142 = Release Notifier(notifier=w34, error in (no error)=w33) -> ()  [unwired: 4 out]
            n143 = Release Queue(queue=w38, error in (no error)=w37) -> ()  [unwired: 1 in, 3 out]
          }
        }
      }
    }
  }
